vi "LimitAlarms.vi"(2 "Value":sgl=3.0 format="%#_13g", 3 "Parameter":sgl=50.0 format="%#_13g") -> (0 "Min":sgl, 1 "Max":sgl)   [LabVIEW 2018]
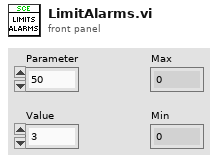
[diagram p1: front panel]
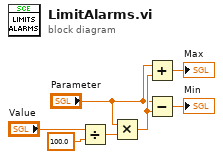
[diagram p0: block diagram]
diagram:
  n1 = Divide(x="Value", y=sgl 100.0) -> (x/y=w3:sgl)
  n2 = Multiply(x="Parameter", y=w3) -> (x*y=w5:sgl)
  n3 = Add(x="Parameter", y=w5) -> (x+y=→"Max":sgl)
  n4 = Subtract(x="Parameter", y=w5) -> (x-y=→"Min":sgl)
